vi "Configure AO Channel.vi"(7 "index":i32, 8 "error in":errorcluster, 10 "config":cluster{"carrier":dbl, "level":dbl}, 11 "fpga session in":refnum<k20>) -> (0 "error out":errorcluster, 3 "fpga session out":refnum<k20>)   [LabVIEW 2018, in "Lock-In Amplifier Example Host.lvlib"]
uses:
  Lock-In Amplifier Example Host.lvlib
  fpga type.ctl
  <vilib>/Utility/error.llb/Error Cluster From Error Code.vi
  <vilib>/rvi/errors/niLvFpgaAdjustHostInterfaceError.vi
  <vilib>/rvi/interface/nirviReadWriteControl/nirviReadWriteControl.xnode
  NiFpgaLv.dll
  <vilib>/rvi/interface/Simulation/niFpgaSimulationCallBeginRW.vi
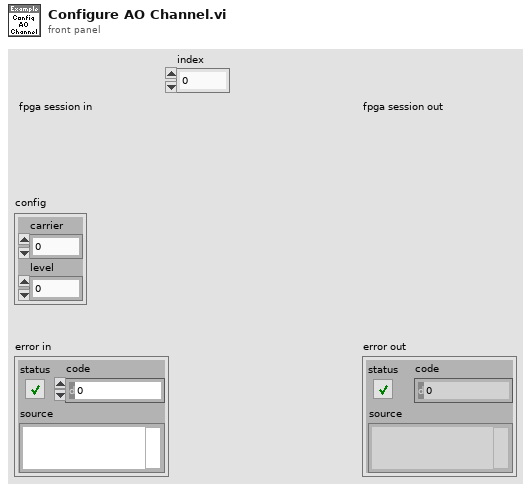
[diagram p1: front panel]
types:
  T1 = typedef "Lock-In Amplifier Example Host.lvlib/fpga type.ctl" = refnum<k20>
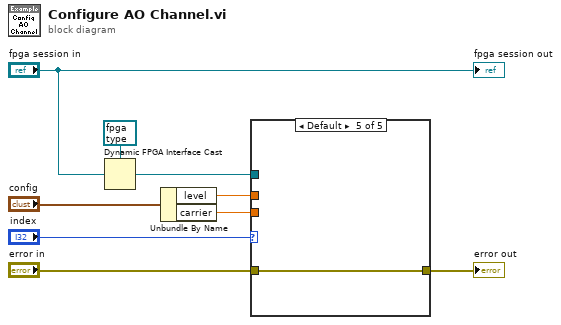
[diagram p0: block diagram]
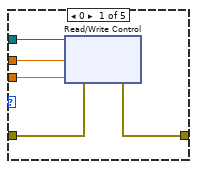
[diagram p2: hidden frame]
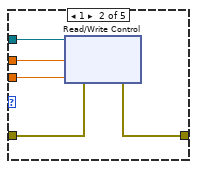
[diagram p3: hidden frame]
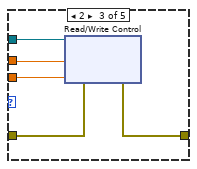
[diagram p4: hidden frame]
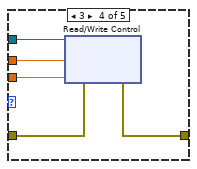
[diagram p5: hidden frame]
diagram:
  n1 = Dynamic FPGA Interface Cast(Session In=T1 refnum ("fpga type"), Type="fpga session in") -> (Session Out=w7:T1)
  n2 = Unbundle By Name("config") -> ("level"=w2:dbl, "carrier"=w1:dbl)
  n3 = case shown="Default" "index" {
    tunnel: w7 -> [w14 w19 w24 w29 _]
    tunnel: "error in" -> [w13 w18 w23 w28 w30]
    tunnel: [w12 w17 w22 w27 w30] -> w3
    tunnel: w2 -> [w11 w16 w21 w26 _]
    tunnel: w1 -> [w10 w15 w20 w25 _]
    frame 0 {
      n4 = xnode "Read/Write Control"("FPGA VI Reference In"=w14, "error in"=w13, "ao.level 0"=w11, "ao.carrier 0"=w10) -> ("error out"=w12:errorcluster)  [unwired: 1 out]
    }
    frame 1 {
      n5 = xnode "Read/Write Control"("FPGA VI Reference In"=w19, "error in"=w18, "ao.level 1"=w16, "ao.carrier 1"=w15) -> ("error out"=w17:errorcluster)  [unwired: 1 out]
    }
    frame 2 {
      n6 = xnode "Read/Write Control"("FPGA VI Reference In"=w24, "error in"=w23, "ao.level 2"=w21, "ao.carrier 2"=w20) -> ("error out"=w22:errorcluster)  [unwired: 1 out]
    }
    frame 3 {
      n7 = xnode "Read/Write Control"("FPGA VI Reference In"=w29, "error in"=w28, "ao.level 3"=w26, "ao.carrier 3"=w25) -> ("error out"=w27:errorcluster)  [unwired: 1 out]
    }
    frame Default {
    }
  }
  "error out" <- w3
  "fpga session out" <- "fpga session in"
